vi "Voltage - Finite Input.vi"() -> ()   [LabVIEW 2012]
doc: "This example demonstrates how to acquire a single buffer of voltage measurements using a DAQmx device.\n\nFor instructions on how to connect your signals to the DAQ device, refer to your device documentation."
uses:
  <vilib>/DAQmx/read.llb/DAQmx Read (Analog 1D Wfm NChan NSamp).vi
  <vilib>/DAQmx/create/channels.llb/DAQmx Create Channel (AI-Voltage-Basic).vi
  <vilib>/DAQmx/configure/timing.llb/DAQmx Timing (Sample Clock).vi
  <vilib>/DAQmx/configure/task.llb/DAQmx Configure Logging (TDMS).vi
  <vilib>/DAQmx/configure/trigger.llb/DAQmx Start Trigger (Digital Edge).vi
  <vilib>/DAQmx/configure/trigger.llb/DAQmx Start Trigger (Analog Edge).vi
  <vilib>/DAQmx/configure/trigger.llb/DAQmx Reference Trigger (Digital Edge).vi
  <vilib>/DAQmx/configure/trigger.llb/DAQmx Reference Trigger (Analog Edge).vi
  <vilib>/DAQmx/miscellaneous.llb/DAQmx Fill In Error Info.vi
  <resource>/objmgr/daqmx.rc
panel:
  out "숫자형":i32=3
  in  "Trigger Type":T1(tab)=enum."Digital Start"
  in  "Edge":i32(ring)=10280 items=["Rising"=10280, "Falling"=10171]
  in  "Digital Trigger Source":tag
  in  "Level (V)":dbl format="%0.2f"
  in  "Hysteresis (V)":dbl
  in  "Slope":i32(ring)=10280 items=["Rising"=10280, "Falling"=10171]
  in  "Analog Trigger Source":string="APFI0"
  in  "Digital Ref Trigger Source":tag
  in  "Edge":i32(ring)=10280 items=["Rising"=10280, "Falling"=10171]
  in  "Pre-Trigger Samples":u32
  in  "Analog Ref Trigger Source":string="APFI0"
  in  "Slope":i32(ring)=10280 items=["Rising"=10280, "Falling"=10171]
  in  "Level (V)":dbl format="%0.2f"
  in  "Pre-Trigger Samples":u32
  out "Waveform Graph":waveform(dbl)[](graph)=[{"t0"=timestamp(3527209517.8114386 s since 1904-01-01), "dt"=1.9999999999999944e-06, "Y"=array[5000 elements], "attributes"=variant("NI_ChannelName"=variant(string "Dev4/ai1"), "NI_UnitDescription"=variant(string "Volts"))}]
  in  "TDMS File Path":path
  in  "Number of Samples":i32=5000
  in  "Sample Rate":dbl=500000.0
  in  "Sample Clock Source":tag="OnboardClock"
  in  "Terminal Configuration":i32(ring)=10083 items=["default"=-1, "RSE"=10083, "NRSE"=10078, "Differential"=10106, "Pseudodifferential"=12529]
  in  "Max Voltage":dbl=10.0
  in  "Min Voltage":dbl=-10.0
  in  "Physical Channel":tag="Dev4/ai1"
  out "Actual Sample Rate":dbl=500000.0 format="%0.2f"
  in  "Logging Mode":i32(ring)=10231 items=["Off"=10231, "Log and Read"=15842]
  # "Channel Settings"
  # "Acquired Data"
  # "Timing Settings"
  # "Trigger Settings"
  # "Logging Settings"
  # "To configure and use a start trigger you must have the necessary tab selected above.  Not all hardware supports triggering--refer to your device documentation for more info."
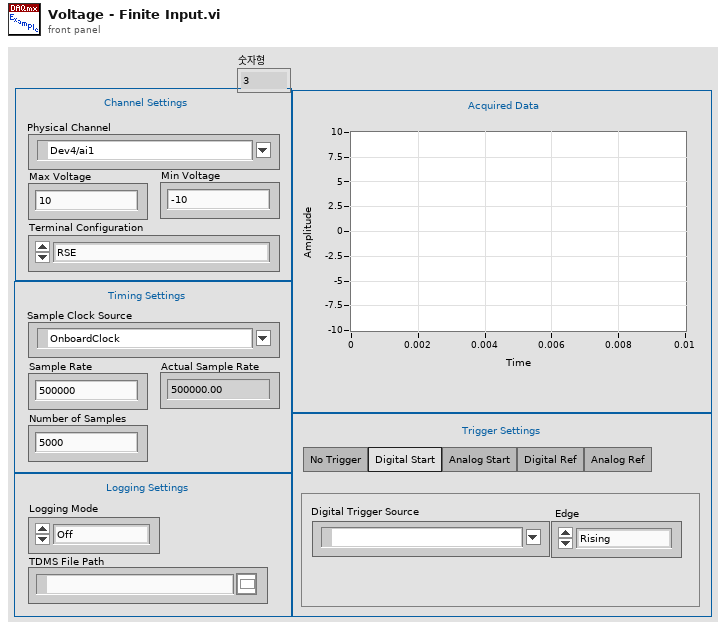
[diagram p1: front panel]
types:
  T1 = enum32{"No Trigger", "Digital Start", "Analog Start", "Digital Ref", "Analog Ref"}
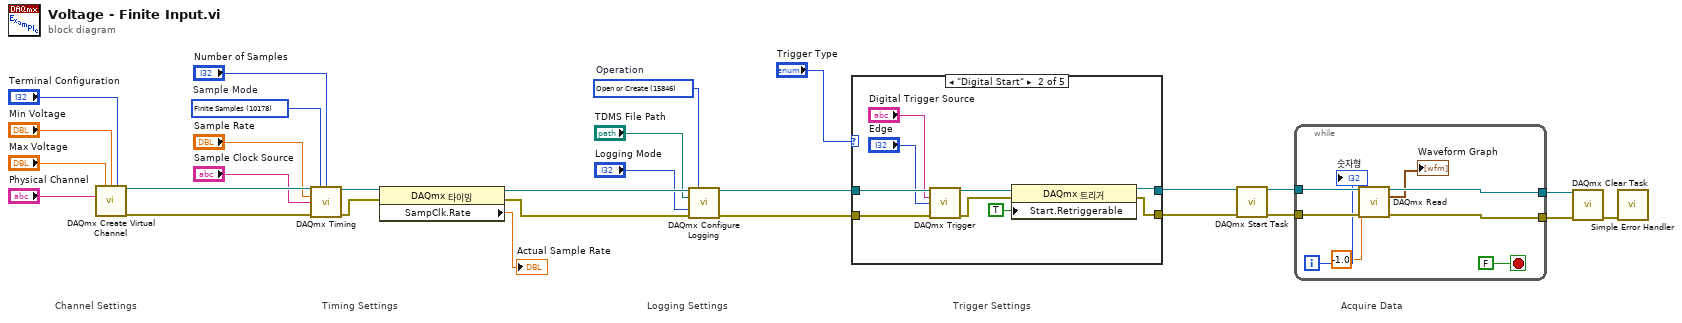
[diagram p0: block diagram]
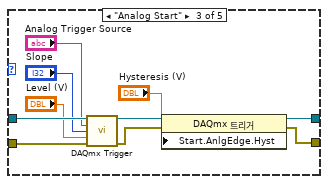
[diagram p3: hidden frame]
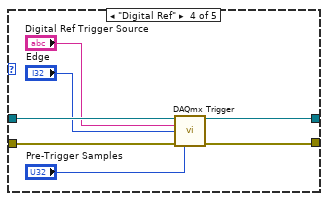
[diagram p4: hidden frame]
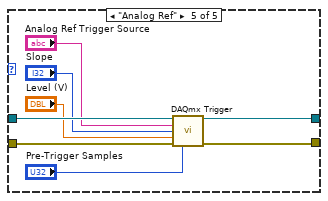
[diagram p5: hidden frame]
diagram:
  w21 = 15846 items=["Open"=10437, "Open or Create"=15846, "Create or Replace"=15847, "Create"=15848]  # Operation
  w26 = 10178 items=["Finite Samples"=10178, "Continuous Samples"=10123, "Hardware Timed Single Point"=12522]  # Sample Mode
  # "Acquire Data"
  # "Trigger Settings"
  # "Timing Settings"
  # "Channel Settings"
  # "Logging Settings"
  n1 = call-poly <vilib>:"DAQmx Create Virtual Channel.vi"("maximum value"="Max Voltage", "minimum value"="Min Voltage", "input terminal configuration"="Terminal Configuration", "physical channels"="Physical Channel") -> ("task out"=w24:refnum<k21>, "error out"=w25:errorcluster)  [unwired: 10 in]
  n2 = call-poly <vilib>:"DAQmx Timing.vi"("task/channels in"=w24, "sample mode"=w26, "samples per channel"="Number of Samples", "rate"="Sample Rate", "source"="Sample Clock Source", "error in"=w25) -> ("task out"=w28:refnum<k21>, "error out"=w27:errorcluster)  [unwired: 8 in]
  n3 = property class="DAQmx 타이밍"(reference=w28, error in=w27) -> (reference out=w23:refnum<k21>, error out=w22:errorcluster, "SampClk.Rate"=→"Actual Sample Rate":dbl)
  n4 = call-poly <vilib>:"DAQmx Configure Logging.vi"("task/channels in"=w23, "operation"=w21, "file path"="TDMS File Path", "logging mode"="Logging Mode", "error in"=w22) -> ("task out"=w20:refnum<k21>, "error out"=w19:errorcluster)  [unwired: 9 in]
  n5 = case shown="\"Digital Start\"" "Trigger Type" {
    tunnel: w20 -> [w30 w39 w49 w56 w64]
    tunnel: w19 -> [w29 w38 w48 w55 w63]
    tunnel: [w30 w34 w46 w54 w58] -> w18
    tunnel: [w29 w33 w45 w53 w59] -> w17
    frame "No Trigger", Default {
    }
    frame "Digital Start" {
      n6 = call-poly <vilib>:"DAQmx Trigger.vi"("task/channels in"=w39, "source"="Digital Trigger Source", "edge"="Edge", "error in"=w38) -> ("task out"=w35:refnum<k21>, "error out"=w32:errorcluster)  [unwired: 10 in]
      n7 = property class="DAQmx 트리거"(reference=w35, error in=w32, "Start.Retriggerable"=TRUE ("시작:추가 옵션:재트리거 가능")) -> (reference out=w34:refnum<k21>, error out=w33:errorcluster)
    }
    frame "Analog Start" {
      n8 = call-poly <vilib>:"DAQmx Trigger.vi"("task/channels in"=w49, "source"="Analog Trigger Source", "slope"="Slope", "level"="Level (V)", "error in"=w48) -> ("task out"=w44:refnum<k21>, "error out"=w43:errorcluster)  [unwired: 9 in]
      n9 = property class="DAQmx 트리거"(reference=w44, error in=w43, "Start.AnlgEdge.Hyst"="Hysteresis (V)") -> (reference out=w46:refnum<k21>, error out=w45:errorcluster)
    }
    frame "Digital Ref" {
      n10 = call-poly <vilib>:"DAQmx Trigger.vi"("task/channels in"=w56, "source"="Digital Ref Trigger Source", "edge"="Edge", "error in"=w55, "pretrigger samples per channel"="Pre-Trigger Samples") -> ("task out"=w54:refnum<k21>, "error out"=w53:errorcluster)  [unwired: 9 in]
    }
    frame "Analog Ref" {
      n11 = call-poly <vilib>:"DAQmx Trigger.vi"("task/channels in"=w64, "source"="Analog Ref Trigger Source", "slope"="Slope", "level"="Level (V)", "error in"=w63, "pretrigger samples per channel"="Pre-Trigger Samples") -> ("task out"=w58:refnum<k21>, "error out"=w59:errorcluster)  [unwired: 8 in]
    }
  }
  n12 = call <vilib>:"DAQmx Start Task.vi"("task/channels in"=w18, "error in"=w17) -> ("task out"=w16:refnum<k21>, "error out"=w15:errorcluster)  [unwired: 12 in]
  n13 = while {
    tunnel: w16 -> [w72]
    tunnel: w15 -> [w71]
    tunnel: [w70] -> w14
    tunnel: [w69] -> w13
    i -> [w67]
    stop <- FALSE stop-if-true
    n14 = call-poly <vilib>:"DAQmx Read.vi"("task/channels in"=w72, "timeout"=-1.0, "error in"=w71) -> ("task out"=w70:refnum<k21>, "data"=→"Waveform Graph":waveform(dbl)[], "error out"=w69:errorcluster)  [unwired: 10 in]
    "숫자형" <- w67
  }
  n15 = call <vilib>:"DAQmx Clear Task.vi"("task in"=w14, "error in"=w13) -> ("error out"=w12:errorcluster)  [unwired: 13 in]
  n16 = call <vilib>:"Simple Error Handler.vi"("error in (no error)"=w12) -> ()  [unwired: 4 in, 5 out]
